vi "OldLockinToDAQSMOConfig.vi"(9 "sampling info":cluster{"Fs":dbl, "#s":dbl}, 10 "AO Configuration":T11, 11 "AI Configuration":T7) -> (3 "DAQ_Manager.setDAQConfig":T1 {"DAQmx.AI.config"."input terminal configuration" items=["default"=-1, "RSE"=10083, "NRSE"=10078, "Differential"=10106, "Pseudodifferential"=12529]; "DAQmx.AI.config"."AI.Coupling" items=["AC"=10045, "DC"=10050]; "DAQmx.AO.config"."output terminal configuration" items=["Default"=-1, "RSE"=10083, "Differential"=10106, "Pseudodifferential"=12529]})   [LabVIEW 2016]
uses:
  DAQmx.AO/Typedefs/AO.Terminal-enum.ctl
  DAQmx.AO/DAQmx.AO.lvclass
  DAQmx.AI/Typedefs/AI.Terminal-enum.ctl
  DAQmx.AI/DAQmx.AI.lvclass
  DAQmx.AO/Typedefs/DAQmx.AO_Config.ctl
  DAQmx.AI/Typedefs/AI.Coupling-enum.ctl
  DAQmx.AI/Typedefs/DAQmx.AI_Config.ctl
  Typedefs/PrivateEvents--DAQ_Manager.setDAQConfig.ctl
  DAQ_Manager.lvclass
  Typedefs/446xAO-enum.ctl
  Typedefs/AO.config-cluster.ctl
  Typedefs/AO.config-array.ctl
  Typedefs/AI.coupling-enum.ctl
  Typedefs/446xAI-enum.ctl
  Typedefs/AI.config-cluster.ctl
  Typedefs/AI.config-array.ctl
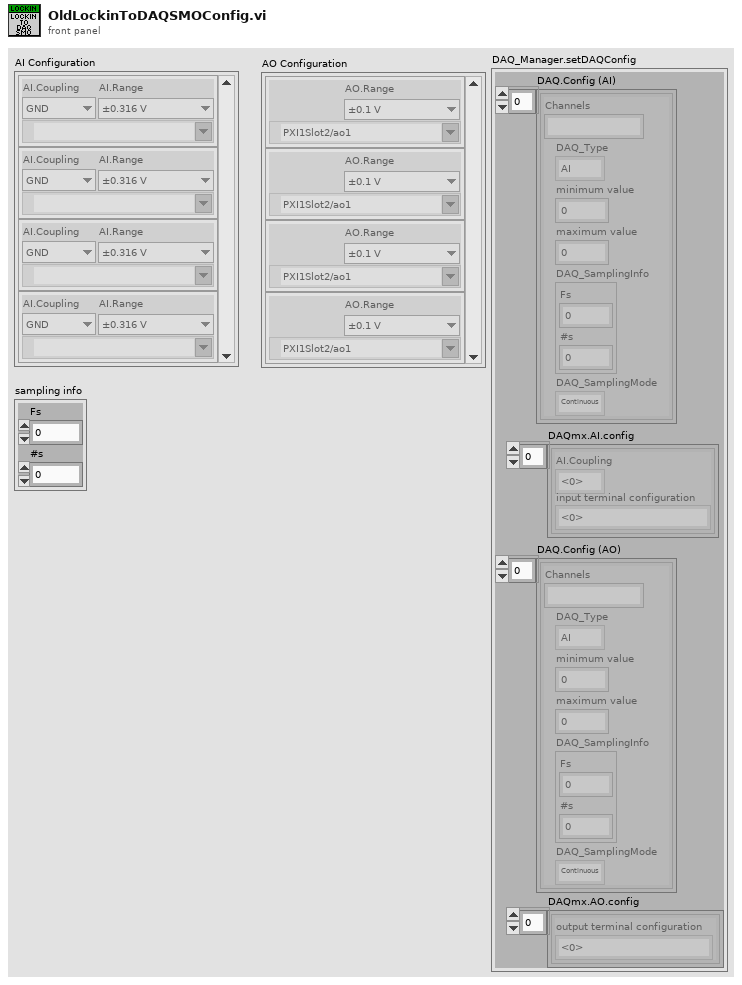
[diagram p1: front panel]
types:
  T1 = typedef "DAQ_Manager.lvclass/PrivateEvents--DAQ_Manager.setDAQConfig.ctl" = cluster{"DAQ.Config (AI)":cluster{"Channels":string, "DAQ_Type":enum16{"AI", "AO"}, "minimum value":dbl, "maximum value":dbl, "DAQ_SamplingInfo":cluster{"Fs":dbl, "#s":i32}, "DAQ_SamplingMode":enum16{"Continuous", "Finite"}}[], "DAQmx.AI.config":T2[], "DAQ.Config (AO)":cluster{"Channels":string, "DAQ_Type":enum16{"AI", "AO"}, "minimum value":dbl, "maximum value":dbl, "DAQ_SamplingInfo":cluster{"Fs":dbl, "#s":i32}, "DAQ_SamplingMode":enum16{"Continuous", "Finite"}}[], "DAQmx.AO.config":T5[]}
  T2 = typedef "DAQmx.AI.lvclass/DAQmx.AI_Config.ctl" = cluster{"AI.Coupling":T3, "input terminal configuration ":T4}
  T3 = typedef "DAQmx.AI.lvclass/AI.Coupling-enum.ctl" = i32
  T4 = typedef "DAQmx.AI.lvclass/AI.Terminal-enum.ctl" = i32
  T5 = typedef "DAQmx.AO.lvclass/DAQmx.AO_Config.ctl" = cluster{"output terminal configuration":T6}
  T6 = typedef "DAQmx.AO.lvclass/AO.Terminal-enum.ctl" = i32
  T7 = typedef "AI.config-array.ctl" = T8[]
  T8 = typedef "AI.config-cluster.ctl" = cluster{"AI.Coupling":T9, "AI.channels":tag, "AI.Range":T10}
  T9 = typedef "AI.coupling-enum.ctl" = enum16{"AC", "DC", "GND"}
  T10 = typedef "446xAI-enum.ctl" = enum16{"±0.316 V", "±1.00 V", "±3.16 V", "±10.0 V", "±31.6 V", "±42.4 V"}
  T11 = typedef "AO.config-array.ctl" = T12[]
  T12 = typedef "AO.config-cluster.ctl" = cluster{"AO.Range":T13, "AO.channels":tag}
  T13 = typedef "446xAO-enum.ctl" = enum16{"±0.1 V", "±1.0 V", "±10.0 V"}
  T14 = cluster{"Channels":string, "DAQ_Type":enum16{"AI", "AO"}, "minimum value":dbl, "maximum value":dbl, "DAQ_SamplingInfo":cluster{"Fs":dbl, "#s":i32}, "DAQ_SamplingMode":enum16{"Continuous", "Finite"}}[]
  T15 = cluster{"Channels":string, "DAQ_Type":enum16{"AI", "AO"}, "minimum value":dbl, "maximum value":dbl, "DAQ_SamplingInfo":cluster{"Fs":dbl, "#s":i32}, "DAQ_SamplingMode":enum16{"Continuous", "Finite"}}
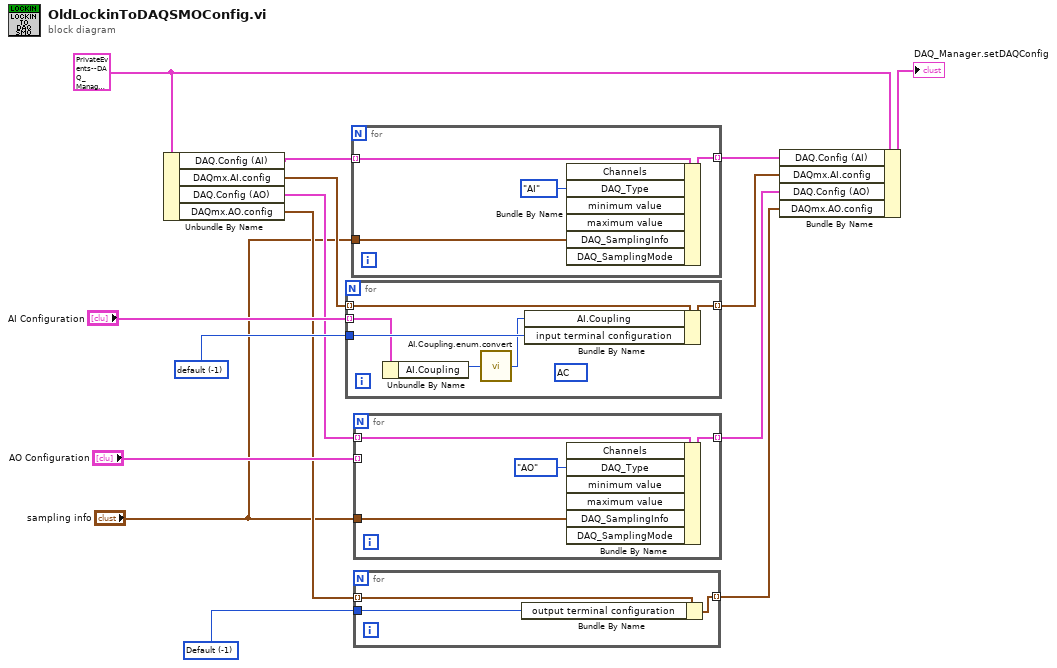
[diagram p0: block diagram]
diagram:
  w3 = T1 {"DAQ.Config (AI)"=[{"Channels"="", "DAQ_Type"=enum."AI", "minimum value"=0.0, "maximum value"=0.0, "DAQ_SamplingInfo"={"Fs"=0.0, "#s"=0}, "DAQ_SamplingMode"=enum."Continuous"}], "DAQmx.AI.config"=[{"AI.Coupling"=10045, "input terminal configuration "=-1}], "DAQ.Config (AO)"=[{"Channels"="", "DAQ_Type"=enum."AI", "minimum value"=0.0, "maximum value"=0.0, "DAQ_SamplingInfo"={"Fs"=0.0, "#s"=0}, "DAQ_SamplingMode"=enum."Continuous"}], "DAQmx.AO.config"=[{"output terminal configuration"=-1}]} ("DAQ_Manager.setDAQConfig")
  w13 = T4 -1 items=["default"=-1, "RSE"=10083, "NRSE"=10078, "Differential"=10106, "Pseudodifferential"=12529] ("input terminal configuration")
  w12 = T6 -1 items=["Default"=-1, "RSE"=10083, "Differential"=10106, "Pseudodifferential"=12529] ("output terminal configuration")
  n1 = Unbundle By Name(w3) -> ("DAQ.Config (AI)"=w5:T14, "DAQmx.AI.config"=w6:T2[], "DAQ.Config (AO)"=w8:T14, "DAQmx.AO.config"=w10:T5[])
  n2 = for {
    tunnel: w6 -> [w21] mode=indexing
    tunnel: [w16] -> w7 mode=indexing
    tunnel: w13 -> [w20]
    tunnel: "AI Configuration" -> [w19] mode=indexing
    (unwired) T3 10045 items=["AC"=10045, "DC"=10050] ("AI.Coupling")
    n3 = Unbundle By Name(w19) -> ("AI.Coupling"=w18:T9)
    n4 = call "AI.Coupling.enum.convert.vi"("AI.Coupling"=w18) -> ("Numeric"=w17:i32)
    n5 = Bundle By Name(cluster=w21, "AI.Coupling"=w17, "input terminal configuration"=w20) -> (w16:T2)
  }
  n6 = for {
    tunnel: w5 -> [w25] mode=indexing
    tunnel: [w24] -> w1 mode=indexing
    tunnel: "sampling info" -> [w22]
    n7 = Bundle By Name(cluster=w25, "DAQ_Type"=enum16{"AI", "AO"}."AI", "DAQ_SamplingInfo"=w22) -> (w24:T15)  [unwired: 4 in]
  }
  n8 = for {
    tunnel: w8 -> [w29] mode=indexing
    tunnel: [w28] -> w9 mode=indexing
    tunnel: "AO Configuration" -> [_] mode=indexing
    tunnel: "sampling info" -> [w26]
    n9 = Bundle By Name(cluster=w29, "DAQ_Type"=enum16{"AI", "AO"}."AO", "DAQ_SamplingInfo"=w26) -> (w28:T15)  [unwired: 4 in]
  }
  n10 = for {
    tunnel: w10 -> [w32] mode=indexing
    tunnel: [w31] -> w11 mode=indexing
    tunnel: w12 -> [w30]
    n11 = Bundle By Name(cluster=w32, "output terminal configuration"=w30) -> (w31:T5)
  }
  n12 = Bundle By Name(cluster=w3, "DAQ.Config (AI)"=w1, "DAQmx.AI.config"=w7, "DAQ.Config (AO)"=w9, "DAQmx.AO.config"=w11) -> (→"DAQ_Manager.setDAQConfig":T1)
